vi "Convert I-V.vi"(8 "error in":errorcluster, 11 "File Path":path) -> (0 "error out":errorcluster, 3 "Output File Path":path)   [LabVIEW 2021, in "Point Contact Model.lvclass"]
uses:
  Libraries/Utilities/Model/BTK/dIdV State/Point Contact Model.lvclass
panel:
  in  "Voltmeter after preamp":bool=TRUE
  in  "I-V channel index":i32=2
  in  "Suffix":string="iv"
  in  "New data channel names":string[](array[string])=["V", "I", "dIdV", "T"]
  out "Number of scans in file":i32
  in  "Preamp gain":dbl=5.0 format="%#_6f"
  in  "Current range":dbl=0.001 format="%#_6pA"
  in  "Lock-in Vout":dbl=0.02 format="%#_6pV"
  out "Scans in file":i32
  in  "...to scan":i32=4
  in  "from scan...":i32
  in  "Data channel names":string[](array[string])=["Prema (7) V", "SRS CS580 (COM4) I", "SRS 830 (10) X", "Cryo-Con 32 (12) A"]
  in  "Measurement technique":T1(ring)=enum."Lock-in dV/dI"
  # "V"
  # "I"
  # "dIdV"
  # "T"
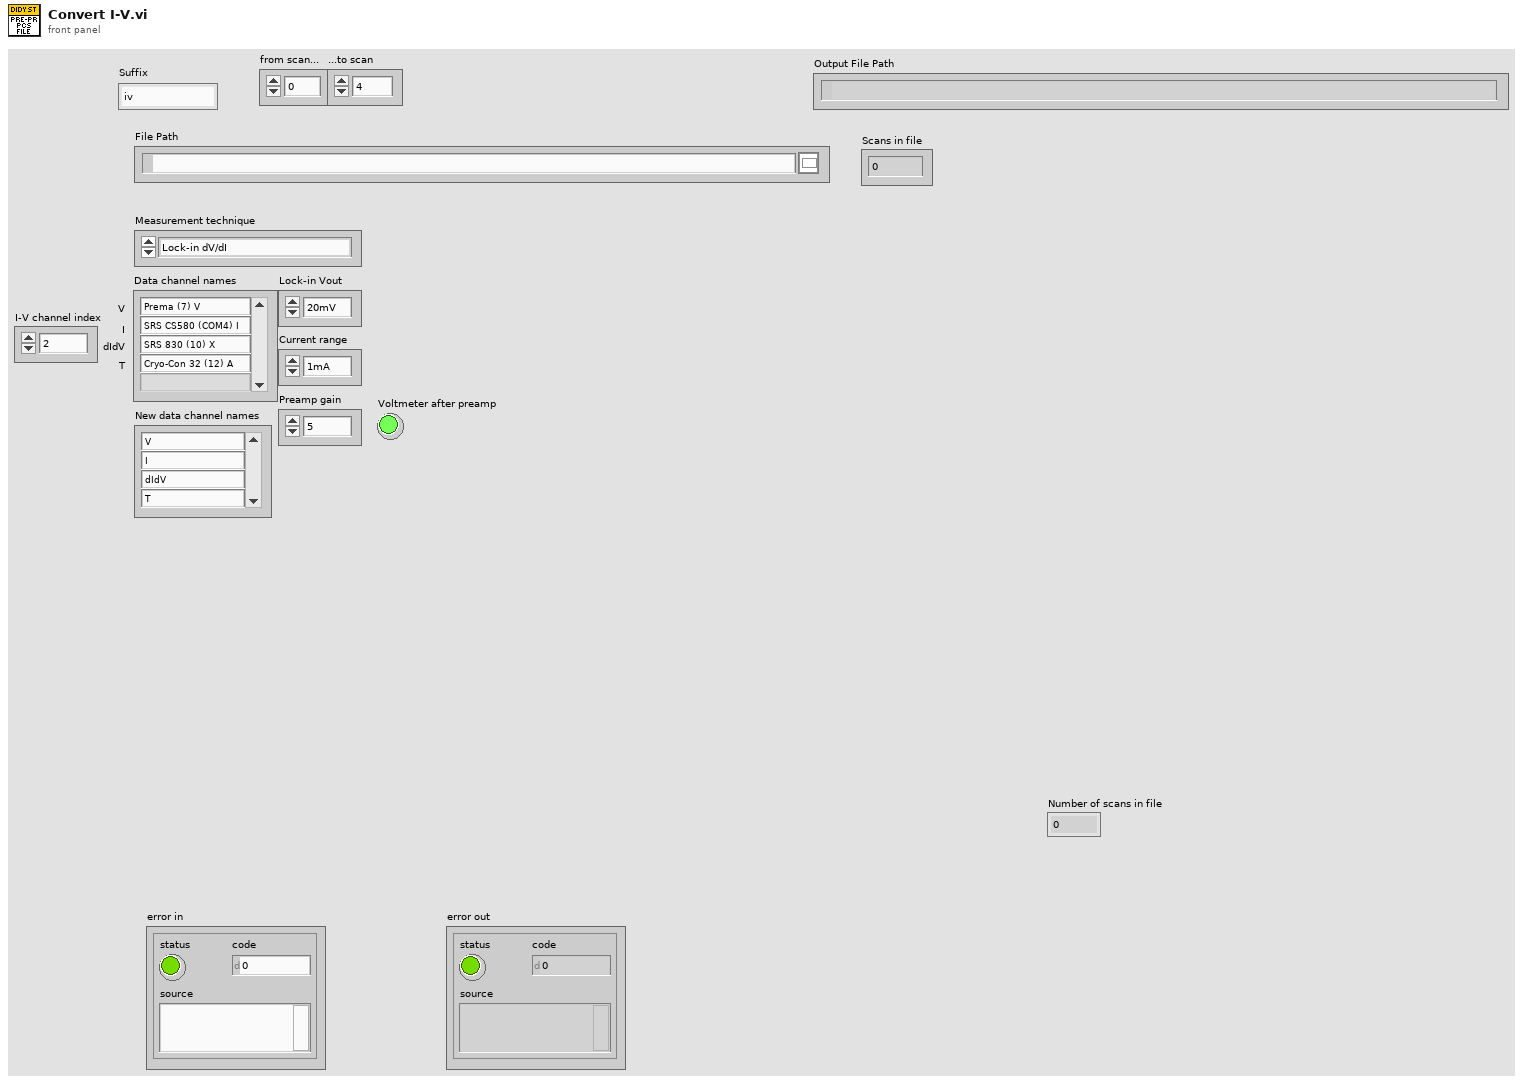
[diagram p1: front panel]
types:
  T1 = enum16{"", "Lock-in dV/dI", "Keithley 6221/2182 "}
  T2 = enum16{"open", "open or create", "create or replace", "create", "open (read-only)"}
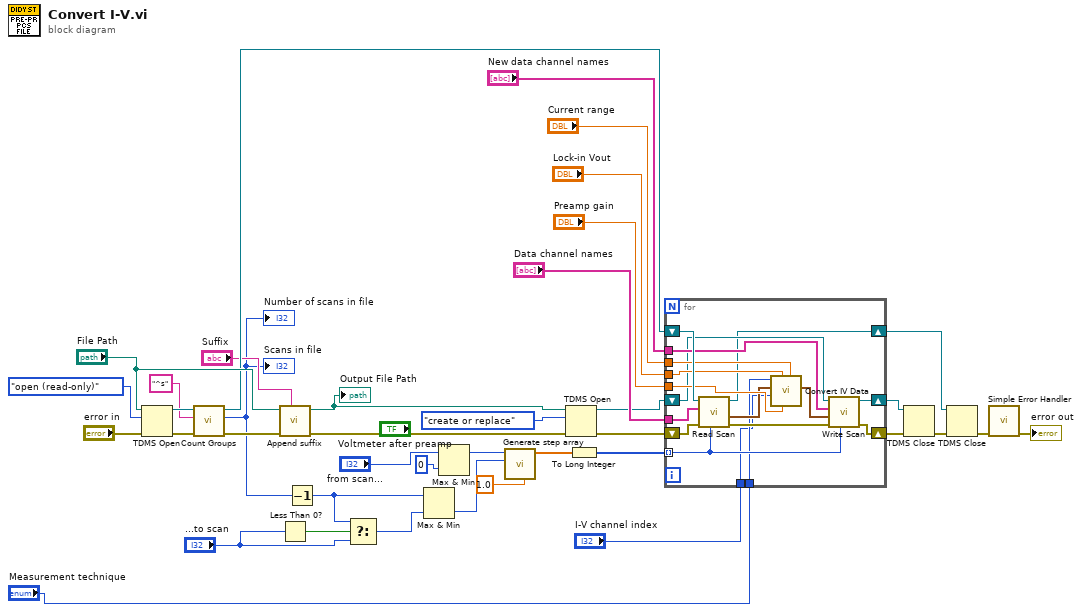
[diagram p0: block diagram]
diagram:
  n1 = TDMS Open(8:"error in", 10:T2."open (read-only)" ("operation (0:open)"), 11:"File Path") -> (0:w22:errorcluster, 3:w38:refnum<k34>)  [unwired: 4 in]
  n2 = call "Count Groups.vi"("error in"=w22, "regular expression"="^s", "tdms file"=w38) -> ("error out"=w13:errorcluster, "Count"=w4:i32, "tdms file out"=w24:refnum<k34>)  [unwired: 5 in, 1 out]
  "Scans in file" <- w4
  "Number of scans in file" <- w4
  n3 = call "Append suffix.vi"("Suffix"="Suffix", "error in (no error)"=w13, "Path"="File Path") -> ("error out"=w16:errorcluster, "Path out"=w17:path)  [unwired: 7 in]
  "Output File Path" <- w17
  n4 = Less Than 0?(x="...to scan") -> (x < 0?=w32:bool)
  n5 = Decrement(x=w4) -> (x-1=w3:i32)
  n6 = Select(t=w3, s=w32, f="...to scan") -> (s? t:f=w30:i32)
  n7 = Max & Min(x=w3, y=w30) -> (min(x,y)=w27:i32)  [unwired: 1 out]
  n8 = Max & Min(x="from scan...", y=0) -> (max(x,y)=w28:i32)  [unwired: 1 out]
  n9 = call "Generate step array.vi"("Step"=1.0, "End"=w27, "Start"=w28) -> ("Steps"=w26:dbl[])  [unwired: 8 in]
  n10 = TDMS Open(8:w16, 10:T2."create or replace" ("operation (0:open)"), 11:w17) -> (0:w12:errorcluster, 3:w14:refnum<k34>)  [unwired: 4 in]
  n11 = To Long Integer(number=w26) -> (32bit integer=w25:i32[])
  n12 = for {
    tunnel: w25 -> [w52] mode=indexing
    shift-right: [w42] -> w8
    shift-left: w24 -> [w53]
    tunnel: "Data channel names" -> [w56]
    shift-right: [w50] -> w11
    shift-left: w12 -> [w55]
    tunnel: "New data channel names" -> [w51]
    tunnel: "Preamp gain" -> [w49]
    tunnel: "Lock-in Vout" -> [w48]
    tunnel: "Current range" -> [w47]
    shift-right: [w43] -> w10
    shift-left: w14 -> [w44]
    tunnel: "Measurement technique" -> [w41]
    tunnel: "I-V channel index" -> [w40]
    n13 = call "Read Scan.vi"("Scan number"=w52, "error in"=w55, "Data channel names"=w56, "tdms file in"=w53) -> ("error out"=w54:errorcluster, "Data channels"=w46:waveform(dbl)[], "tdms file out"=w42:refnum<k34>)  [unwired: 5 in]
    n14 = call "Convert IV Data.vi"("Current range"=w47, "Preamp gain"=w49, "Lock-in Vout"=w48, "I-V index"=w40, "Data in"=w46, "Measurement technique"=w41) -> ("Data out"=w45:waveform(dbl)[])  [unwired: 5 in]
    n15 = call "Write Scan.vi"("Scan number"=w52, "error in"=w54, "Data channels"=w45, "Data channel names"=w51, "tdms file in"=w44) -> ("error out"=w50:errorcluster, "tdms file out"=w43:refnum<k34>)  [unwired: 5 in]
  }
  n16 = TDMS Close(8:w11, 11:w10) -> (0:w9:errorcluster)  [unwired: 1 out]
  n17 = TDMS Close(8:w9, 11:w8) -> (0:w7:errorcluster)  [unwired: 1 out]
  n18 = call <vilib>:"Simple Error Handler.vi"("error in (no error)"=w7) -> ("error out"=→"error out":errorcluster)  [unwired: 4 in, 4 out]
